vi "Read Mutation Type.vi"(8 "error in (no error)":errorcluster, 11 "GA in":refnum<class "GA.lvclass">) -> (0 "error out":errorcluster, 2 "Mutation Type":T1, 3 "GA out":refnum<class "GA.lvclass">)   [LabVIEW 2013, in "GA.lvclass"]
uses:
  GA.lvclass
  Controls/Mutation Type.ctl
  GA.lvclass/GA.ctl
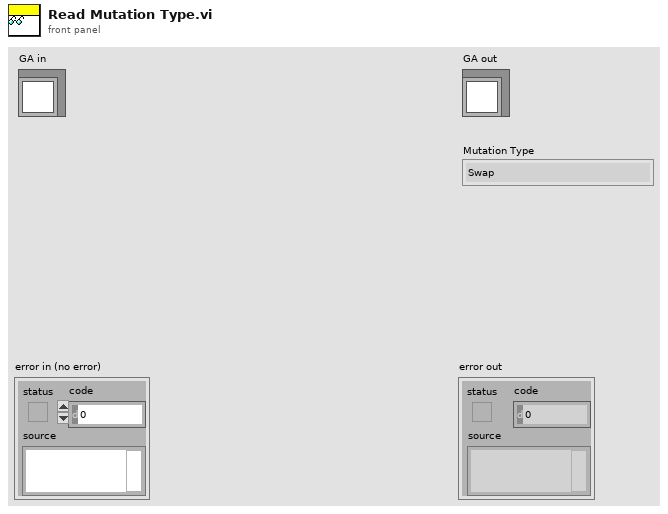
[diagram p1: front panel]
types:
  T1 = typedef "GA.lvclass/Mutation Type.ctl" = enum16{"Swap", "Non-Redundant Swap", "Insert", "Shift", "Shuflle", "Inversion", "SA", "IRH3T", "JO4M Swap", "MO4J Swap", "SPT JO4M", "SPT MO4J", "LCTJ Swap", "Low's Mutation", "ND Mutation"}
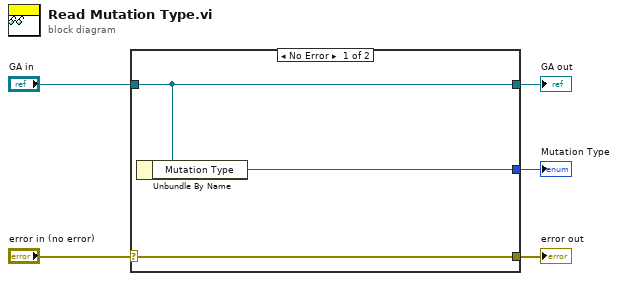
[diagram p0: block diagram]
diagram:
  n1 = case shown="No Error" "error in (no error)" {
    selector: "error in (no error)" -> [w8 w9]
    tunnel: [w8 w9] -> w4
    tunnel: [w7 w10] -> w2
    tunnel: "GA in" -> [w7 w10]
    tunnel: [w6 _] -> w1
    frame No Error {
      n2 = Unbundle By Name(w7) -> ("Mutation Type"=w6:T1)
    }
    frame Error {
    }
  }
  "error out" <- w4
  "GA out" <- w2
  "Mutation Type" <- w1
